vi "Pre Allocate Method Results.vi"(11 "LUnit Test Case In":refnum<class "LUnit Test Case.lvclass">) -> (3 "LUnit Test Case Out":refnum<class "LUnit Test Case.lvclass">)   [LabVIEW 2020, in "LUnit Test Case.lvclass"]
uses:
  LUnit Test Case.lvclass
  Result Types/Case Result/Test Case Result.lvlib
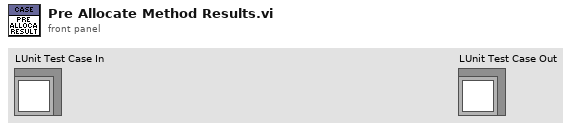
[diagram p1: front panel]
types:
  T1 = typedef "Test Case Result.lvlib/Test Case Result.ctl" = map{string, T2}
  T2 = typedef "Method Result.lvlib/Method Result.ctl" = cluster{"Test Case":string, "Test Method Name":string, "Status":T3, "Assertion Results":T4[], "Execution time":dbl, "Result String":string}
  T3 = typedef "Assertion Result.lvlib/Status.ctl" = enum16{"Pass", "Fail", "Error", "Skipped", "Setup Error", "Broken", "Teardown Error"}
  T4 = typedef "Assertion Result.lvlib/Assertion Result.ctl" = cluster{"Status":T3, "Message":string, "Description":string, "Assertion Type":T5}
  T5 = typedef "Assertion Result.lvlib/Assertion Type.ctl" = enum16{"None", "Pass", "Fail", "Skip", "Pass if Equal", "Fail if Equal", "Pass if Error", "Fail if Error", "Pass if", "Fail if"}
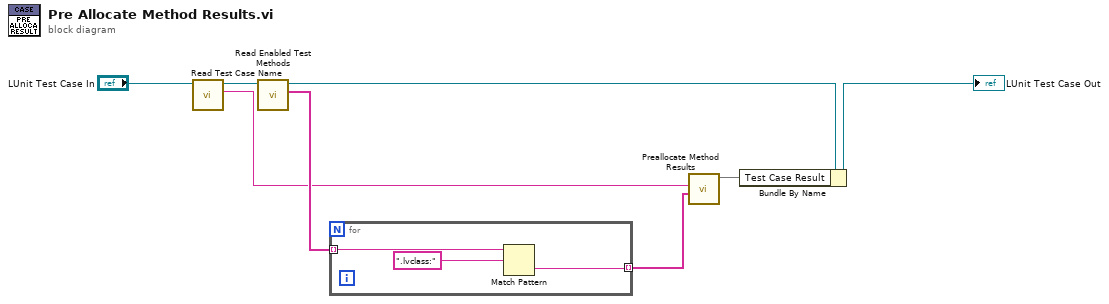
[diagram p0: block diagram]
diagram:
  n1 = call "Read Test Case Name.vi"("LUnit Test Case In"="LUnit Test Case In") -> ("Test Case Name"=w2:string, "LUnit Test Case Out"=w6:refnum<class "LUnit Test Case.lvclass">)  [unwired: 9 in]
  n2 = call "Read Enabled Test Methods.vi"("LUnit Test Case In"=w6) -> ("Names"=w5:string[], "LUnit Test Case Out"=w8:refnum<class "LUnit Test Case.lvclass">)  [unwired: 8 in, 1 out]
  n3 = for {
    tunnel: w5 -> [w10] mode=indexing
    tunnel: [w9] -> w1 mode=indexing
    n4 = Match Pattern(string=w10, regular expression=".lvclass:") -> (after substring=w9:string)  [unwired: 1 in, 3 out]
  }
  n5 = call "Preallocate Method Results.vi"("Test Methods"=w1, "Test Case"=w2) -> ("Test Case Result out"=w3:T1)  [unwired: 9 in]
  n6 = Bundle By Name(cluster=w8, "Test Case Result"=w3) -> (→"LUnit Test Case Out":refnum<class "LUnit Test Case.lvclass">)
